vi "WriteData.vi"(8 "Error In":errorcluster, 10 "Data In":u8[](array[numeric]), 11 "Connection In":refnum<k5>) -> (0 "Error Out":errorcluster, 3 "Connection Out":refnum<k5>)   [LabVIEW 2019]
panel:
  out "bytes written":i32
  out "size(s)":i32
  out "length":i32
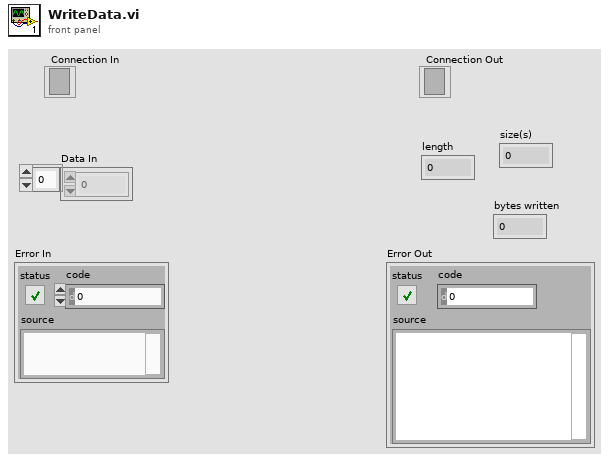
[diagram p1: front panel]
types:
  T1 = enum16{"big-endian, network order", "native, host order", "little-endian"}
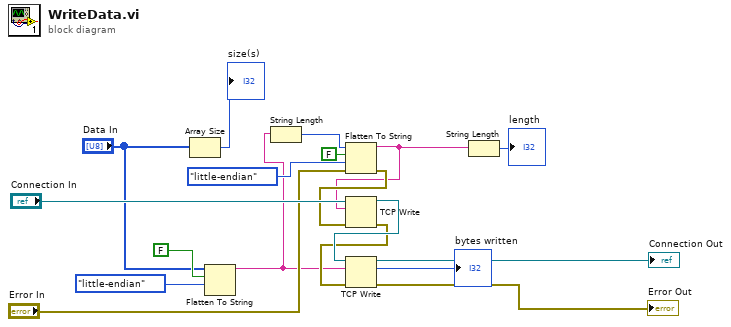
[diagram p0: block diagram]
diagram:
  n1 = Array Size(array="Data In") -> (size(s)=→"size(s)":i32)
  n2 = Flatten To String(anything="Data In", prepend array or string size? (T)=FALSE, byte order (0:big-endian, network order)=T1."little-endian") -> (data string=w4:string)  [unwired: 1 in, 2 out]
  n3 = String Length(string=w4) -> (length=w3:i32)
  n4 = Flatten To String(anything=w3, prepend array or string size? (T)=FALSE, byte order (0:big-endian, network order)=T1."little-endian", error in (no error)="Error In") -> (data string=w7:string, error out=w14:errorcluster)  [unwired: 1 out]
  n5 = TCP Write(connection ID="Connection In", data in=w7, error in (no error)=w14) -> (connection ID out=w17:refnum<k5>, error out=w13:errorcluster)  [unwired: 1 in, 1 out]
  n6 = TCP Write(connection ID=w17, data in=w4, error in (no error)=w13) -> (connection ID out=→"Connection Out":refnum<k5>, bytes written=→"bytes written":i32, error out=→"Error Out":errorcluster)  [unwired: 1 in]
  n7 = String Length(string=w7) -> (length=→"length":i32)
